vi "generate forbidden path error.vi"(8 "error in (no error)":errorcluster, 11 "Data Cluster in":T1) -> (0 "error out":errorcluster)   [LabVIEW 2025, in "Scripting Server.lvlib"]
uses:
  Scripting Server.lvlib
  <vilib>/Utility/error.llb/Error Cluster From Error Code.vi
  <vilib>/ErrorRing/Error Ring.xnode
  Config Data.ctl
  Module Data--cluster.ctl
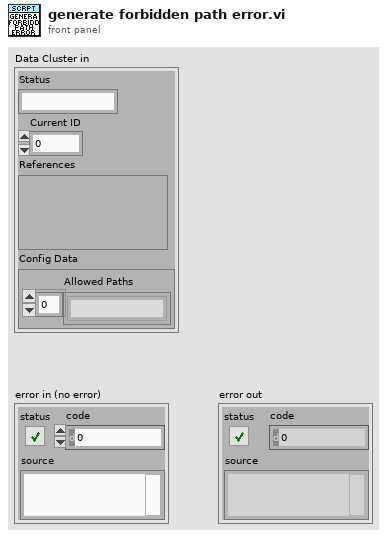
[diagram p1: front panel]
types:
  T1 = typedef "Scripting Server.lvlib/Module Data--cluster.ctl" = cluster{"Status":string, "Current ID":i32, "References":variant, "Config Data":T2}
  T2 = typedef "Scripting Server.lvlib/Config Data.ctl" = cluster{"Allowed Paths":string[]}
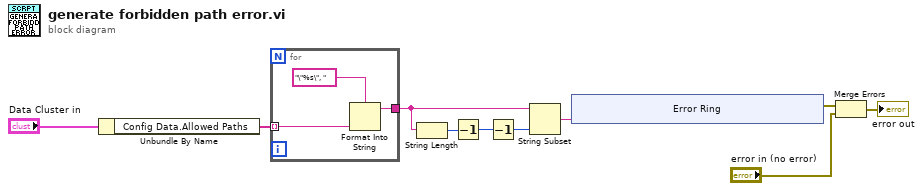
[diagram p0: block diagram]
diagram:
  n1 = Unbundle By Name("Data Cluster in") -> ("Config Data.Allowed Paths"=w4:string[])
  n2 = for {
    tunnel: w4 -> [w11] mode=indexing
    tunnel: [w12] -> w5
    n3 = Format Into String(format string="\"%s\", ", w11) -> (resulting string=w12:string)  [unwired: 2 in, 1 out]
  }
  n4 = String Length(string=w5) -> (length=w7:i32)
  n5 = Decrement(x=w7) -> (x-1=w6:i32)
  n6 = Decrement(x=w6) -> (x-1=w8:i32)
  n7 = String Subset(string=w5, length (rest)=w8) -> (substring=w10:string)  [unwired: 1 in]
  n8 = xnode "Error Ring"("parameter 0"=w10) -> ("error out"=w3:errorcluster)
  n9 = Merge Errors(w3, "error in (no error)") -> (→"error out":errorcluster)
